vi "reset.vi"(8 "error in (no error)":errorcluster, 11 "FgenKeysight in":refnum<class "ArbKeysight.lvclass">) -> (0 "error out":errorcluster, 3 "FgenKeysight out":refnum<class "ArbKeysight.lvclass">)   [LabVIEW 2023, in "ArbKeysight.lvclass"]
doc: "<b>Author:</b> Wolfgang\n<b>Description:</b> This method is used to reset the instrument to a default and known state."
uses:
  ArbKeysight.lvclass
  ArbKeysight.lvclass/ArbKeysight.ctl
  Arb.lvclass
  Driver/Keysight-33500B.lvlib
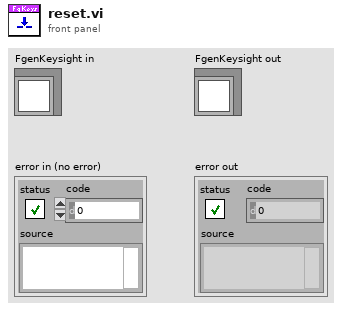
[diagram p1: front panel]
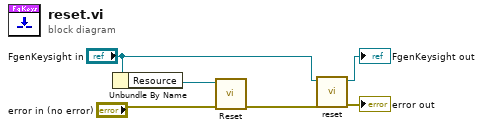
[diagram p0: block diagram]
diagram:
  n1 = Unbundle By Name("FgenKeysight in") -> ("Resource"=w2:refnum<visa-resource-name>)
  n2 = call "Reset.vi"("error in (no error)"="error in (no error)", "VISA resource name"=w2) -> ("error out"=w1:errorcluster)  [unwired: 8 in, 1 out]
  n3 = call-parent "reset.vi"("error in (no error)"=w1, "Instrument in"="FgenKeysight in") -> ("error out"=→"error out":errorcluster, "Instrument out"=→"FgenKeysight out":refnum<class "ArbKeysight.lvclass">)  [unwired: 8 in]
